vi "MLLF_CommandDelimeterSplit.vi"(9 "param 3":string, 10 "param 2":string, 11 "param 1":string) -> (3 "trimmed string":string)   [LabVIEW 2018]
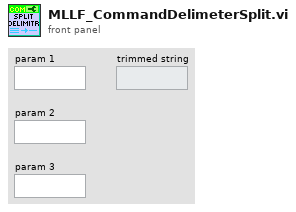
[diagram p1: front panel]
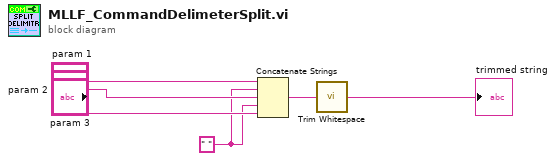
[diagram p0: block diagram]
diagram:
  w1 = " "
  n1 = Concatenate Strings("param 1", w1, "param 2", w1, "param 3") -> (w2:string)
  n2 = call <vilib>:"Trim Whitespace.vi"("string"=w2) -> ("trimmed string"=→"trimmed string":string)  [unwired: 1 in]
